vi "channelStatusSetByName.vi"(7 "Channel names set":T1, 9 "Ch State":T2, 11 "searchString":string) -> (1 "timeTaken":dbl)   [LabVIEW 2022 SP3]
uses:
  ADAM Controls/Channel_State.ctl
  ADAM Controls/Channel_names.ctl
panel:
  # "Sets the status of all channels containing searchString"
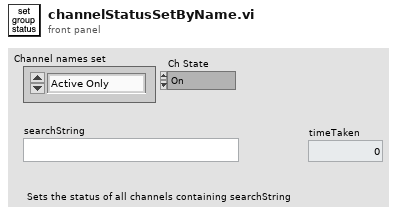
[diagram p1: front panel]
types:
  T1 = typedef "Channel_names.ctl" = enum16{"Active Only", "Active + Off", "All Channels", "Changeable Only", "Always Off", "Always On", "Always Off or On"}
  T2 = typedef "Channel_State.ctl" = enum16{"On", "Off", "Always On", "Always Off"}
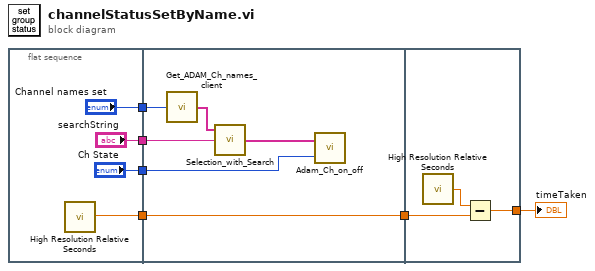
[diagram p0: block diagram]
diagram:
  n1 = flat-sequence {
    tunnel: ["searchString"] -> w6
    tunnel: ["Channel names set"] -> w5
    tunnel: ["Ch State"] -> w4
    tunnel: [w7] -> w3
    tunnel: w6 -> [w15]
    tunnel: w5 -> [w14]
    tunnel: w4 -> [w11]
    tunnel: w3 -> [w13]
    tunnel: [w13] -> w2
    tunnel: w2 -> [w17]
    tunnel: [w19] -> w1
    frame #0 {
      n2 = call <vilib>:"High Resolution Relative Seconds.vi"() -> ("relative seconds"=w7:dbl)
    }
    frame #1 {
      n3 = call "Get_ADAM_Ch_names_client.vi"("Channel names set"=w14) -> ("Ch names"=w16:string[])
      n4 = call "Selection_with_Search.vi"("Search String"=w15, "All Channel Names"=w16) -> ("Item Names"=w12:string[])  [unwired: 1 in]
      n5 = call "Adam_Ch_on_off.vi"("Ch State"=w11, "ADAM Ch Names"=w12) -> ()  [unwired: 1 out]
    }
    frame #2 {
      n6 = call <vilib>:"High Resolution Relative Seconds.vi"() -> ("relative seconds"=w18:dbl)
      n7 = Subtract(x=w18, y=w17) -> (x-y=w19:dbl)
    }
  }
  "timeTaken" <- w1
